vi "Apply Rxn Time.vi"(8 "error in (no error)":errorcluster, 10 "Trxn":dbl, 11 "TTLControl in":refnum<class "TTLController.lvclass">) -> (0 "error out":errorcluster, 3 "TTLControl out":refnum<class "TTLController.lvclass">)   [LabVIEW 2020, in "TTLController.lvclass"]
uses:
  TTLController.lvclass
  TTLController.lvclass/TTLController.ctl
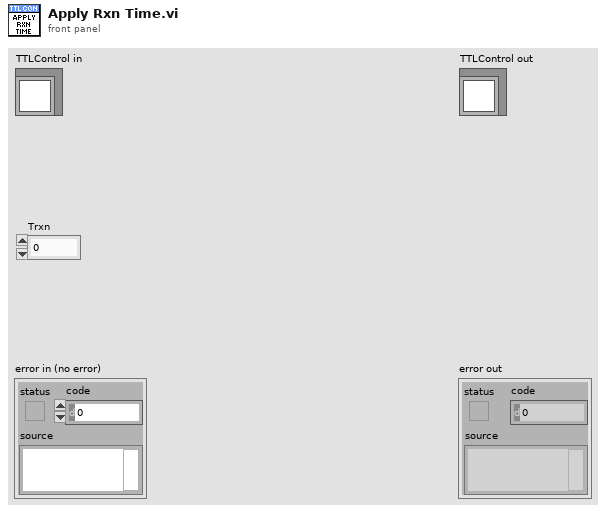
[diagram p1: front panel]
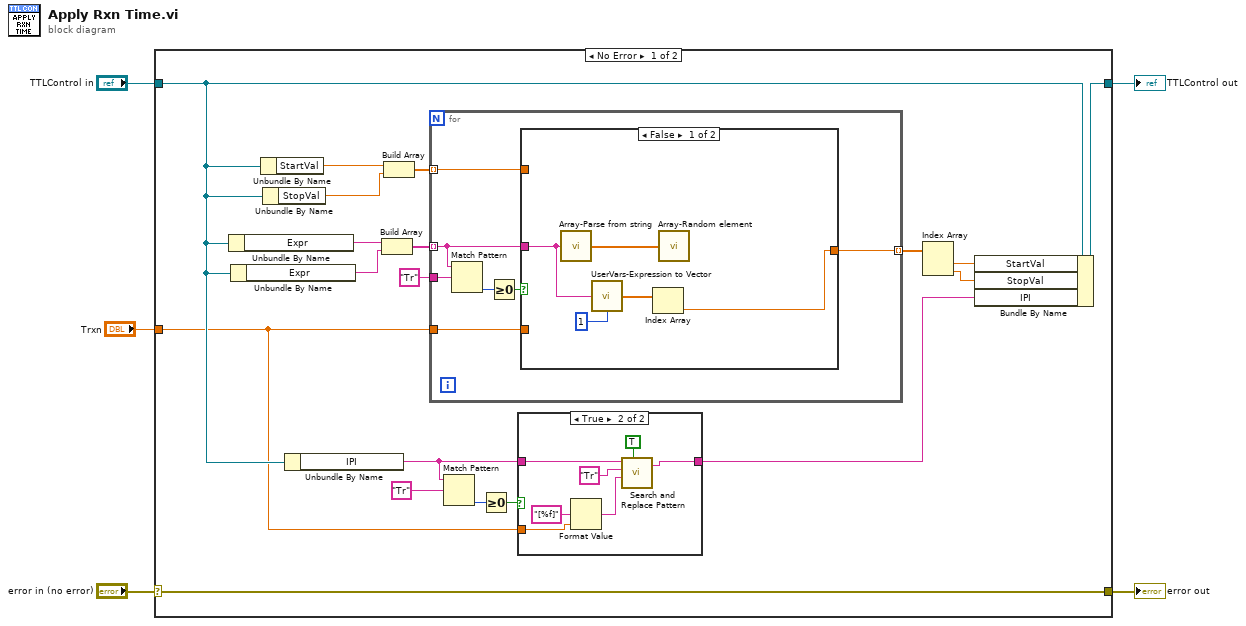
[diagram p0: block diagram]
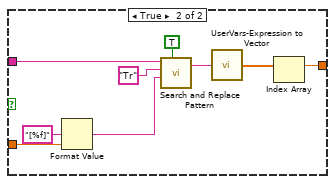
[diagram p3: hidden frame]
diagram:
  n1 = case shown="No Error" "error in (no error)" {
    selector: "error in (no error)" -> [w24 w55]
    tunnel: [w24 w55] -> w4
    tunnel: [w22 w54] -> w2
    tunnel: "TTLControl in" -> [w12 w54]
    tunnel: "Trxn" -> [w6 _]
    frame No Error {
      n2 = Unbundle By Name(w12) -> ("Expr"=w23:string)
      n3 = Unbundle By Name(w12) -> ("Expr"=w20:string)
      n4 = Unbundle By Name(w12) -> ("StartVal"=w15:dbl)
      n5 = Unbundle By Name(w12) -> ("StopVal"=w14:dbl)
      n6 = Unbundle By Name(w12) -> ("IPI"=w9:string)
      n7 = Build Array(w23, w20) -> (w21:string[])
      n8 = Build Array(w15, w14) -> (w13:dbl[])
      n9 = for {
        tunnel: w21 -> [w38] mode=indexing
        tunnel: [w39] -> w19 mode=indexing
        tunnel: "Tr" -> [w37]
        tunnel: w13 -> [w34] mode=indexing
        tunnel: w6 -> [w33]
        n10 = Match Pattern(string=w38, regular expression=w37) -> (offset past match=w36:i32)  [unwired: 1 in, 3 out]
        n11 = Greater Or Equal To 0?(x=w36) -> (x >= 0?=w35:bool)
        n12 = case shown="False" w35 {
          tunnel: [w41 w45] -> w39
          tunnel: w38 -> [w44 w51]
          tunnel: w34 -> [_ _]
          tunnel: w33 -> [_ w53]
          frame False {
            n13 = call "Array-Parse from string.vi"("String"=w44) -> ("Array"=w40:dbl[])  [unwired: 13 in, 1 out]
            n14 = call "UserVars-Expression to Vector.vi"("Expr"=w44, "Nrand"=1) -> ("Values"=w42:dbl[])  [unwired: 12 in, 1 out]
            n15 = Index Array(array=w42) -> (element=w41:dbl)  [unwired: 1 in]
            n16 = call "Array-Random element.vi"("Array"=w40) -> ()  [unwired: 1 in, 2 out]
          }
          frame True {
            n17 = Format Value(format string="[%f]", value (0)=w53) -> (output string=w50:string)  [unwired: 1 in]
            n18 = call <vilib>:"Search and Replace Pattern.vi"("string"=w51, "regular expression (\"\")"="Tr" ("regular expression (\"\")"), "replace string (\"\")"=w50, "replace all? (F)"=TRUE) -> ("result string"=w47:string)  [unwired: 1 in, 1 out]
            n19 = call "UserVars-Expression to Vector.vi"("Expr"=w47) -> ("Values"=w46:dbl[])  [unwired: 13 in, 1 out]
            n20 = Index Array(array=w46) -> (element=w45:dbl)  [unwired: 1 in]
          }
        }
      }
      n21 = Match Pattern(string=w9, regular expression="Tr") -> (offset past match=w10:i32)  [unwired: 1 in, 3 out]
      n22 = Greater Or Equal To 0?(x=w10) -> (x >= 0?=w7:bool)
      n23 = case shown="True" w7 {
        tunnel: w9 -> [w25 w28]
        tunnel: [w25 w27] -> w11
        tunnel: w6 -> [_ w26]
        frame False {
        }
        frame True {
          n24 = Format Value(format string="[%f]", value (0)=w26) -> (output string=w31:string)  [unwired: 1 in]
          n25 = call <vilib>:"Search and Replace Pattern.vi"("string"=w28, "regular expression (\"\")"="Tr" ("regular expression (\"\")"), "replace string (\"\")"=w31, "replace all? (F)"=TRUE) -> ("result string"=w27:string)  [unwired: 1 in, 1 out]
        }
      }
      n26 = Index Array(array=w19) -> (element #1=w18:dbl, element #2=w17:dbl)  [unwired: 2 in]
      n27 = Bundle By Name(cluster=w12, "StartVal"=w18, "StopVal"=w17, "IPI"=w11) -> (w22:refnum<class "TTLController.lvclass">)
    }
    frame Error {
    }
  }
  "error out" <- w4
  "TTLControl out" <- w2
